vi "Remove_duplicate__.vi"(1 "Output String":string) -> (0 "String":string)   [LabVIEW 2010]
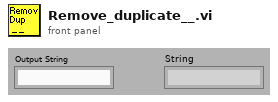
[diagram p1: front panel]
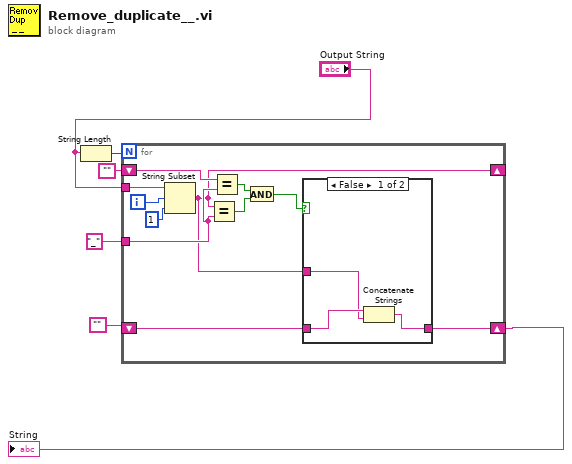
[diagram p0: block diagram]
diagram:
  n1 = String Length(string="Output String") -> (length=w1:i32)
  n2 = for {
    N: w1 -> [_]
    tunnel: "Output String" -> [w15]
    tunnel: "_" -> [w13]
    shift-right: [w7] -> _
    shift-left: "" -> [w14]
    shift-right: [w8] -> w6
    shift-left: "" -> [w9]
    i -> [w16]
    n3 = String Subset(string=w15, offset (0)=w16, length (rest)=1 ("length (rest)")) -> (substring=w7:string)
    n4 = Equal?(x=w7, y=w13) -> (x = y?=w12:bool)
    n5 = Equal?(x=w14, y=w13) -> (x = y?=w11:bool)
    n6 = And(x=w11, y=w12) -> (x .and. y?=w10:bool)
    n7 = case shown="False" w10 {
      tunnel: w9 -> [w20 w21]
      tunnel: [w19 w21] -> w8
      tunnel: w7 -> [w18 _]
      frame False {
        n8 = Concatenate Strings(w20, w18) -> (w19:string)
      }
      frame True {
      }
    }
  }
  "String" <- w6
